vi "TAT_Com_PLC_Simulation.vi"() -> ()   [LabVIEW 2017]
panel:
  out "Array 2":u16[](array[numeric])
  in  "Input From PLC":u16[](array[numeric])
  out "Array":i32[](array[numeric])
  out "PLC STATUS":bool
  in  "error in":errorcluster
  in  "stop":bool
  # "Model Selection\n\n\nCycle Start\n\n\nCycle End\n\n\nCycle result"
  # "PLC Simulator"
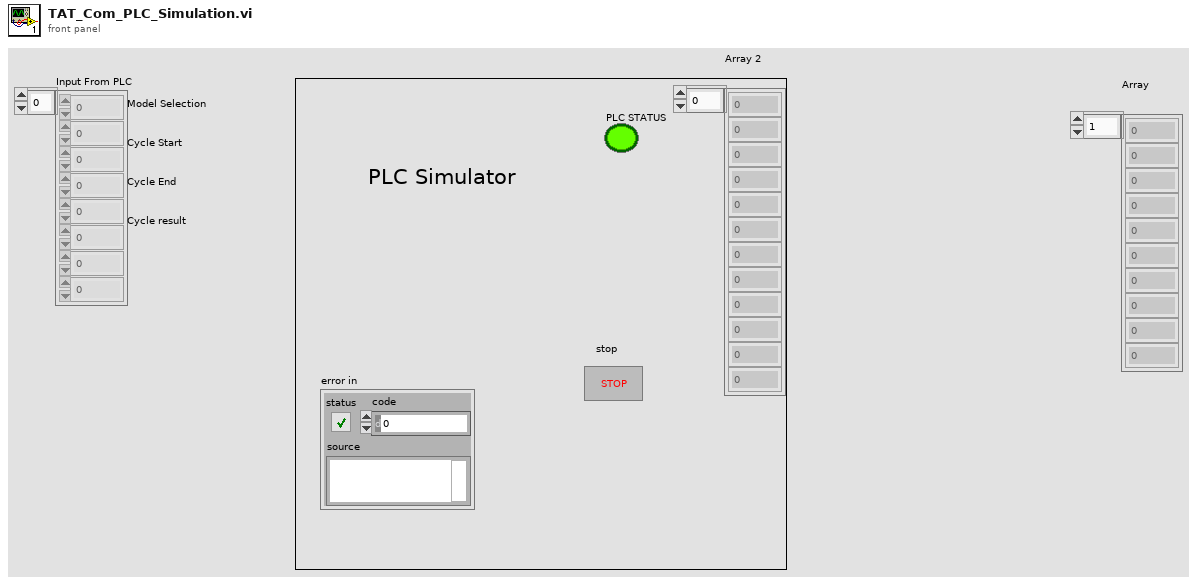
[diagram p1: front panel]
types:
  T1 = enum32{"invalid app kind", "Development System", "Run Time System", "Student Edition", "Embedded LabVIEW", "Evaluation", "Custom"}
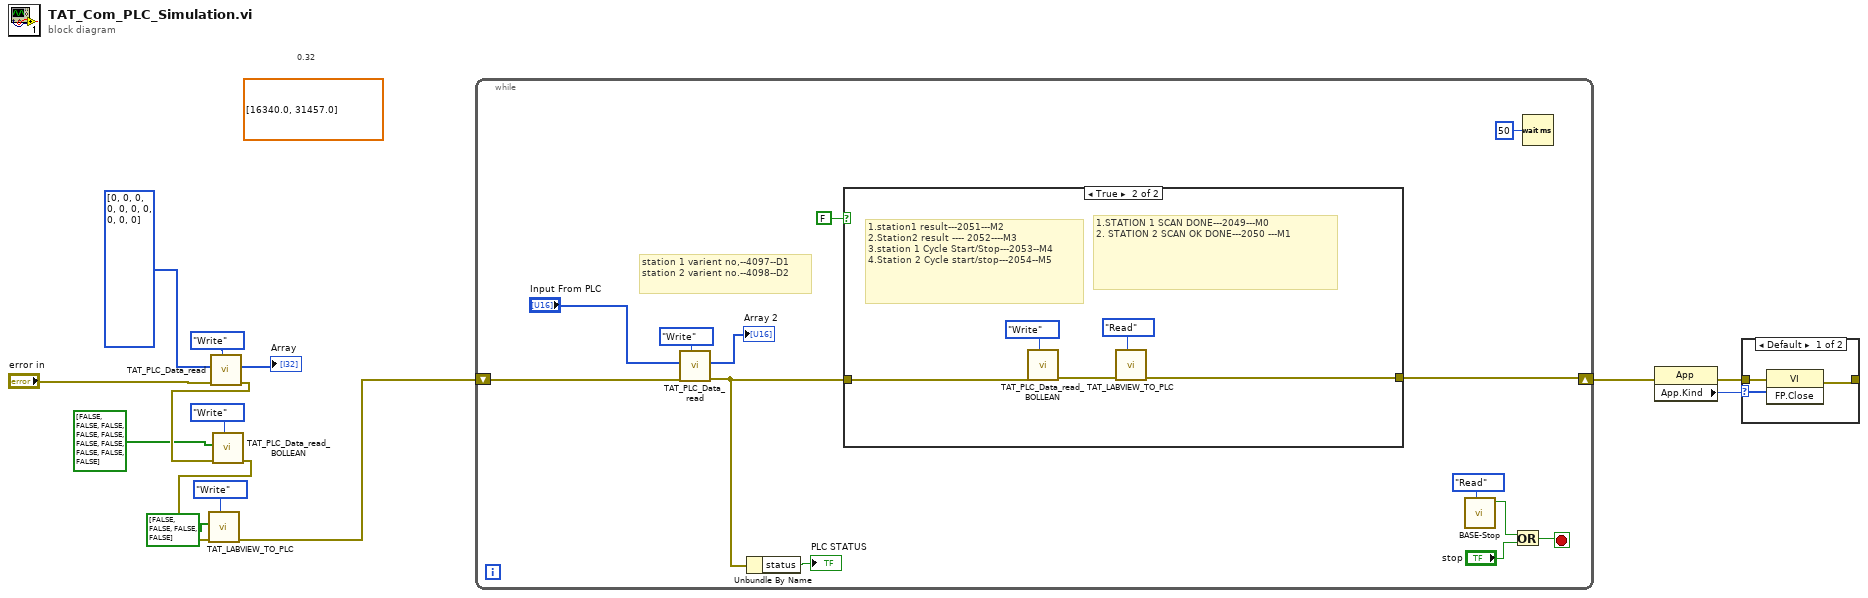
[diagram p0: block diagram]
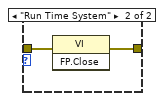
[diagram p3: hidden frame]
diagram:
  (unwired) dbl[] [16340.0, 31457.0] ("register values")
  # "0.32"
  n1 = call "TAT_PLC_Data_read.vi"("Enum"=enum16{"Read", "Write"}."Write", "error in (no error)"="error in", "Array"=i64[] [0, 0, 0, 0, 0, 0, 0, 0, 0, 0] ("Array 3")) -> ("error out"=w7:errorcluster, "Array 2"=→"Array":u16[])  [unwired: 7 in]
  n2 = call "TAT_PLC_Data_read_BOLLEAN.vi"("Enum"=enum16{"Read", "Write"}."Write", "error in (no error)"=w7, "Array"=bool[] [FALSE, FALSE, FALSE, FALSE, FALSE, FALSE, FALSE, FALSE, FALSE, FALSE]) -> ("error out"=w3:errorcluster)  [unwired: 7 in, 1 out]
  n3 = call "TAT_LABVIEW_TO_PLC.vi"("Enum"=enum16{"Read", "Write"}."Write", "error in (no error)"=w3, "Array"=bool[] [FALSE, FALSE, FALSE, FALSE]) -> ("error out"=w4:errorcluster)  [unwired: 7 in, 1 out]
  n4 = while {
    shift-right: [w21] -> w1
    shift-left: w4 -> [w17]
    stop <- w26 stop-if-true
    # "station 1 varient no,--4097--D1\nstation 2 varient no.--4098--D2"
    n5 = call "TAT_PLC_Data_read.vi"("Enum"=enum16{"Read", "Write"}."Write", "error in (no error)"=w17, "Array"="Input From PLC") -> ("error out"=w22:errorcluster, "Array 2"=→"Array 2":u16[])  [unwired: 7 in]
    n6 = Unbundle By Name(w22) -> ("status"=→"PLC STATUS":bool)
    n7 = case shown="True" FALSE {
      tunnel: w22 -> [w28 w33]
      tunnel: [w28 w29] -> w21
      frame False {
      }
      frame True {
        # "1.STATION 1 SCAN DONE---2049---M0\n2. STATION 2 SCAN OK DONE---2050 ---M1"
        # "1.station1 result---2051---M2\n2.Station2 result ---- 2052----M3\n3.station 1 Cycle Start/Stop---2053--M4\n4.Station 2 Cycle start/stop---2054--M5"
        n8 = call "TAT_PLC_Data_read_BOLLEAN.vi"("Enum"=enum16{"Read", "Write"}."Write", "error in (no error)"=w33) -> ("error out"=w30:errorcluster)  [unwired: 8 in, 1 out]
        n9 = call "TAT_LABVIEW_TO_PLC.vi"("Enum"=enum16{"Read", "Write"}."Read", "error in (no error)"=w30) -> ("error out"=w29:errorcluster)  [unwired: 8 in, 1 out]
      }
    }
    n10 = call "BASE-Stop.vi"("Enum"=enum16{"Read", "Write"}."Read") -> ("Stop"=w19:bool)  [unwired: 10 in]
    n11 = Or(x=w19, y="stop") -> (x .or. y?=w26:bool)
    n12 = Wait (ms)(milliseconds to wait=u32 50) -> ()  [unwired: 1 out]
  }
  n13 = property class="App"(error in=w1) -> (error out=w13:errorcluster, "App.Kind"=w14:T1)  [unwired: 1 in, 1 out]
  n14 = case shown="Default" w14 {
    tunnel: w13 -> [w35 w37]
    tunnel: [w34 w36] -> _
    frame Default {
      n15 = invoke class="VI" method="FP.Close"(error in=w35) -> (error out=w34:errorcluster)  [unwired: 2 in, 2 out]
    }
    frame "Run Time System" {
      n16 = invoke class="VI" method="FP.Close"(error in=w37) -> (error out=w36:errorcluster)  [unwired: 2 in, 2 out]
    }
  }
